vi "Read detector calibrations.vi"(4 "Contrast B":sgl=40.0, 5 "Brightness B":sgl=40.0, 6 "Contrast A":sgl=26.0, 7 "Brightness A":sgl=40.0, 11 "Path":path) -> (3 "Latest 8-bit coefficients":sgl[][](array[numeric]))   [LabVIEW 2018]
uses:
  <vilib>/Utility/file.llb/Read Delimited Spreadsheet (string).vi
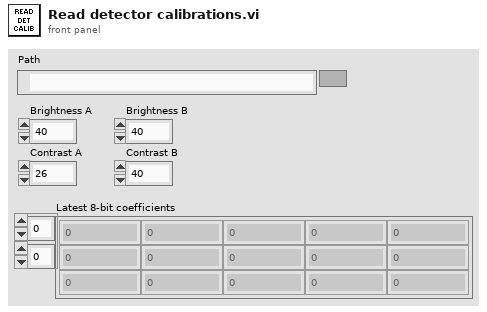
[diagram p1: front panel]
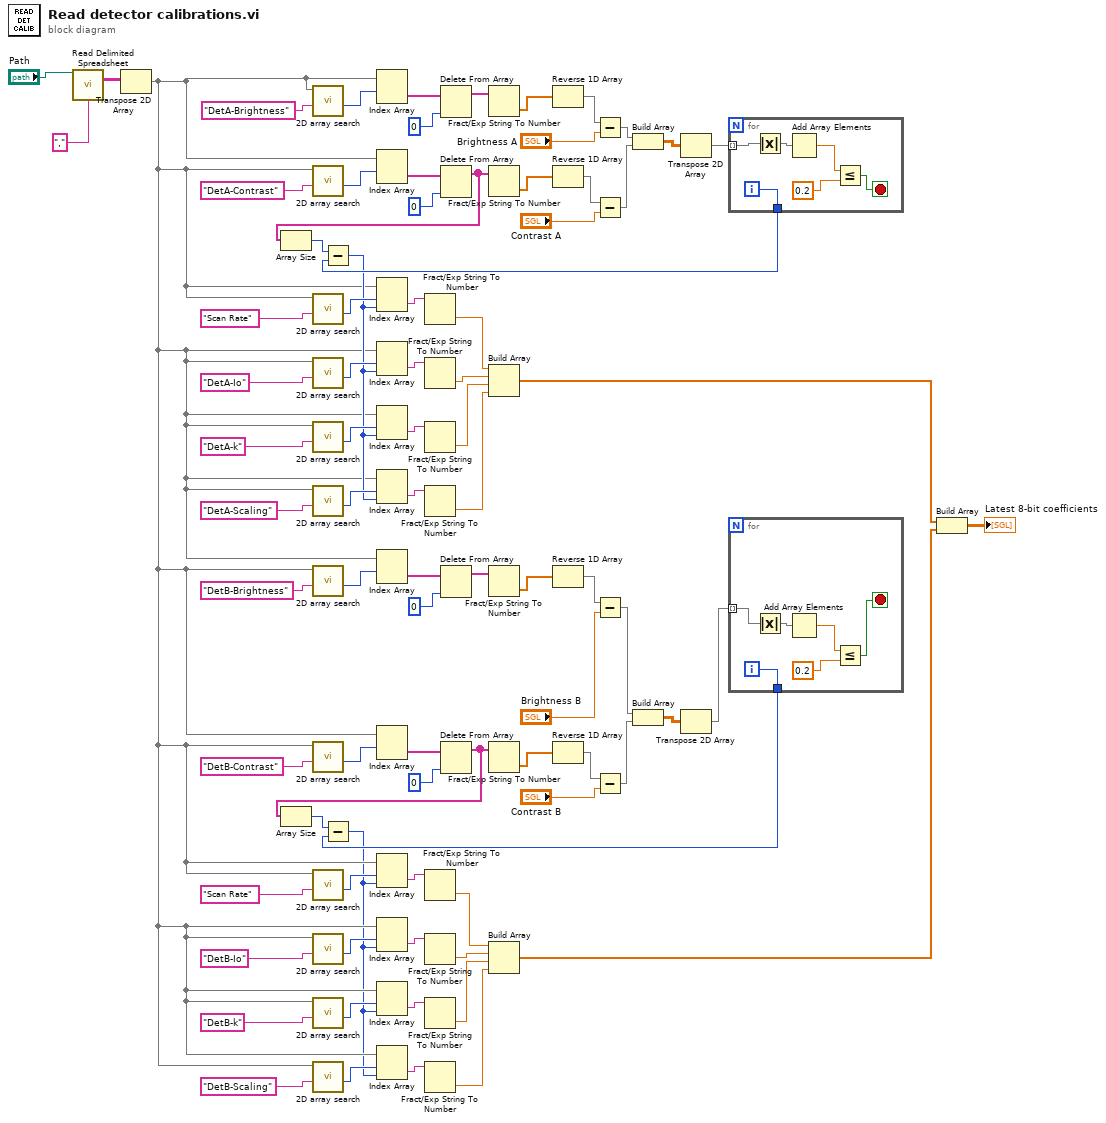
[diagram p0: block diagram]
diagram:
  n1 = call-poly <vilib>:"Read Delimited Spreadsheet.vi"("file path (dialog if empty)"="Path", "delimiter (\\t)"="," ("delimiter (\\t)")) -> ("all rows"=w1:string[][])  [unwired: 8 in, 5 out]
  n2 = Transpose 2D Array(2D array=w1) -> (transposed array=w6:string[][])
  n3 = call "2D array search.vi"("Search For"="DetA-Brightness", "Input Array"=w6) -> ("Row"=w85:i32)  [unwired: 7 in, 2 out]
  n4 = call "2D array search.vi"("Search For"="DetA-Contrast", "Input Array"=w6) -> ("Row"=w78:i32)  [unwired: 7 in, 2 out]
  n5 = call "2D array search.vi"("Search For"="Scan Rate", "Input Array"=w6) -> ("Row"=w22:i32)  [unwired: 7 in, 2 out]
  n6 = call "2D array search.vi"("Search For"="DetA-Io", "Input Array"=w6) -> ("Row"=w66:i32)  [unwired: 7 in, 2 out]
  n7 = call "2D array search.vi"("Search For"="DetA-k", "Input Array"=w6) -> ("Row"=w69:i32)  [unwired: 7 in, 2 out]
  n8 = call "2D array search.vi"("Search For"="DetA-Scaling", "Input Array"=w6) -> ("Row"=w12:i32)  [unwired: 7 in, 2 out]
  n9 = call "2D array search.vi"("Search For"="DetB-Brightness", "Input Array"=w6) -> ("Row"=w39:i32)  [unwired: 7 in, 2 out]
  n10 = call "2D array search.vi"("Search For"="DetB-Contrast", "Input Array"=w6) -> ("Row"=w47:i32)  [unwired: 7 in, 2 out]
  n11 = call "2D array search.vi"("Search For"="Scan Rate", "Input Array"=w6) -> ("Row"=w16:i32)  [unwired: 7 in, 2 out]
  n12 = call "2D array search.vi"("Search For"="DetB-Io", "Input Array"=w6) -> ("Row"=w57:i32)  [unwired: 7 in, 2 out]
  n13 = call "2D array search.vi"("Search For"="DetB-k", "Input Array"=w6) -> ("Row"=w54:i32)  [unwired: 7 in, 2 out]
  n14 = call "2D array search.vi"("Search For"="DetB-Scaling", "Input Array"=w6) -> ("Row"=w9:i32)  [unwired: 7 in, 2 out]
  n15 = Index Array(array=w6, index (row)=w85) -> (element=w83:string[])  [unwired: 1 in]
  n16 = Index Array(array=w6, index (row)=w78) -> (element=w29:string[])  [unwired: 1 in]
  n17 = Index Array(array=w6, index (row)=w39) -> (element=w41:string[])  [unwired: 1 in]
  n18 = Index Array(array=w6, index (row)=w47) -> (element=w45:string[])  [unwired: 1 in]
  n19 = Delete From Array(array=w83, index=0) -> (array with subset deleted=w81:string[])  [unwired: 1 in, 1 out]
  n20 = Delete From Array(array=w29, index=0) -> (array with subset deleted=w28:string[])  [unwired: 1 in, 1 out]
  n21 = Array Size(array=w28) -> (size(s)=w27:i32)
  n22 = Delete From Array(array=w41, index=0) -> (array with subset deleted=w43:string[])  [unwired: 1 in, 1 out]
  n23 = Delete From Array(array=w45, index=0) -> (array with subset deleted=w24:string[])  [unwired: 1 in, 1 out]
  n24 = Array Size(array=w24) -> (size(s)=w25:i32)
  n25 = Fract/Exp String To Number(string=w81) -> (number=w74:dbl[])  [unwired: 4 out]
  n26 = Fract/Exp String To Number(string=w28) -> (number=w75:dbl[])  [unwired: 4 out]
  n27 = Fract/Exp String To Number(string=w43) -> (number=w49:dbl[])  [unwired: 4 out]
  n28 = Fract/Exp String To Number(string=w24) -> (number=w48:dbl[])  [unwired: 4 out]
  n29 = Reverse 1D Array(array=w74) -> (reversed array=w33:dbl[])
  n30 = Reverse 1D Array(array=w75) -> (reversed array=w32:dbl[])
  n31 = Reverse 1D Array(array=w49) -> (reversed array=w31:dbl[])
  n32 = Reverse 1D Array(array=w48) -> (reversed array=w30:dbl[])
  n33 = Subtract(x=w33, y="Brightness A") -> (x-y=w70:dbl[])
  n34 = Subtract(x=w32, y="Contrast A") -> (x-y=w71:dbl[])
  n35 = Subtract(x=w31, y="Brightness B") -> (x-y=w53:dbl[])
  n36 = Subtract(x=w30, y="Contrast B") -> (x-y=w52:dbl[])
  n37 = Build Array(w70, w71) -> (w73:dbl[][])
  n38 = Build Array(w53, w52) -> (w50:dbl[][])
  n39 = Transpose 2D Array(2D array=w73) -> (transposed array=w72:dbl[][])
  n40 = Transpose 2D Array(2D array=w50) -> (transposed array=w51:dbl[][])
  n41 = for {
    tunnel: w72 -> [w91] mode=indexing
    tunnel: [w87] -> w26
    i -> [w87]
    stop <- w88 stop-if-true
    n42 = Absolute Value(x=w91) -> (abs(x)=w86:dbl[])
    n43 = Add Array Elements(numeric array=w86) -> (sum=w90:dbl)
    n44 = Less Or Equal?(x=w90, y=0.2) -> (x <= y?=w88:bool)
  }
  n45 = Subtract(x=w27, y=w26) -> (x-y=w10:i32)
  n46 = Index Array(array=w6, index (row)=w22, index (col)=w10) -> (element=w20:string)
  n47 = Index Array(array=w6, index (row)=w66, index (col)=w10) -> (element=w65:string)
  n48 = Index Array(array=w6, index (row)=w69, index (col)=w10) -> (element=w64:string)
  n49 = Index Array(array=w6, index (row)=w12, index (col)=w10) -> (element=w14:string)
  n50 = Fract/Exp String To Number(string=w20) -> (number=w19:dbl)  [unwired: 4 out]
  n51 = Fract/Exp String To Number(string=w65) -> (number=w63:dbl)  [unwired: 4 out]
  n52 = Fract/Exp String To Number(string=w64) -> (number=w62:dbl)  [unwired: 4 out]
  n53 = Fract/Exp String To Number(string=w14) -> (number=w11:dbl)  [unwired: 4 out]
  n54 = Build Array(w19, w63, w62, w11) -> (w36:dbl[])
  n55 = for {
    tunnel: w51 -> [w97] mode=indexing
    tunnel: [w93] -> w23
    i -> [w93]
    stop <- w94 stop-if-true
    n56 = Absolute Value(x=w97) -> (abs(x)=w92:dbl[])
    n57 = Add Array Elements(numeric array=w92) -> (sum=w96:dbl)
    n58 = Less Or Equal?(x=w96, y=0.2) -> (x <= y?=w94:bool)
  }
  n59 = Subtract(x=w25, y=w23) -> (x-y=w5:i32)
  n60 = Index Array(array=w6, index (row)=w16, index (col)=w5) -> (element=w18:string)
  n61 = Index Array(array=w6, index (row)=w57, index (col)=w5) -> (element=w58:string)
  n62 = Index Array(array=w6, index (row)=w54, index (col)=w5) -> (element=w59:string)
  n63 = Index Array(array=w6, index (row)=w9, index (col)=w5) -> (element=w7:string)
  n64 = Fract/Exp String To Number(string=w18) -> (number=w15:dbl)  [unwired: 4 out]
  n65 = Fract/Exp String To Number(string=w58) -> (number=w60:dbl)  [unwired: 4 out]
  n66 = Fract/Exp String To Number(string=w59) -> (number=w61:dbl)  [unwired: 4 out]
  n67 = Fract/Exp String To Number(string=w7) -> (number=w4:dbl)  [unwired: 4 out]
  n68 = Build Array(w15, w60, w61, w4) -> (w35:dbl[])
  n69 = Build Array(w36, w35) -> (→"Latest 8-bit coefficients":dbl[][])
